vi "Periodic Tasks.vi"(8 "error in":errorcluster) -> ()   [LabVIEW 2014]
doc: "This VI runs in parallel to other tasks. It can contain as many user-defined periodic loops as you need. These can carry out PID or other sorts of timed response."
uses:
  <vilib>/Rock Robotics/WPI/Joystick/WPI_JoystickGetSetRefNum.vi
  <vilib>/Rock Robotics/WPI/RobotDrive/WPI_RobotDriveGetSetRefNum.vi
  <vilib>/Rock Robotics/Network Tables/SD Read Numeric Array.vi
  Robot Global Data.vi
  <vilib>/Rock Robotics/Network Tables/SD Write Numeric Array.vi
  <vilib>/Rock Robotics/Network Tables/SD Write Number.vi
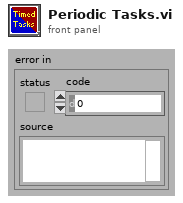
[diagram p1: front panel]
types:
  T1 = cluster{"[0]":dbl, "[1]":dbl, "[2]":dbl, "[3]":dbl, "[4]":dbl, "[5]":dbl, "[6]":dbl, "[7]":dbl, "[8]":dbl}
  T2 = typedef "WPI_JoystickDevRef.ctl" = cluster{"Device":T3}
  T3 = typedef "WPI_JoystickDeviceEnum.ctl" = enum16{"USB 0", "USB 1", "USB 2", "USB 3", "USB 4", "USB 5"}
  T4 = typedef "WPI_RobotDriveDevRef.ctl" = cluster{"DevStatus":errorcluster, "Motors[]":T5[], "Square Inputs":bool, "Max Output":dbl}
  T5 = typedef "WPI_MotorControlDeviceRef.ctl" = cluster{"DeviceStatus":errorcluster, "Type":T6, "PWM":cluster{"Controller":T7, "PWM Channel":T8, "DeadBand":T9}, "CAN":cluster{"Device Number":u8, "Control Mode":T10, "Semaphore":T11, "Max Vout":dbl, "TalonSRX Control Mode":T12}, "Invert":bool, "TransformRef":T13, "InvTransformRef":T13}
  T6 = typedef "WPI_MotorControlType.ctl" = enum16{"PWM", "CAN", "CANTalonSRX"}
  T7 = typedef "FPGA_TypedefDigitalModule.ctl" = enum16{"Controller 1"}
  T8 = typedef "FPGA_DIOPWMChannel.ctl" = enum8{"PWM 0", "PWM 1", "PWM 2", "PWM 3", "PWM 4", "PWM 5", "PWM 6", "PWM 7", "PWM 8", "PWM 9", "PWM MXP 0", "PWM MXP 1", "PWM MXP 2", "PWM MXP 3", "PWM MXP 4", "PWM MXP 5", "PWM MXP 6", "PWM MXP 7", "PWM MXP 8", "PWM MXP 9", "Invalid"}
  T9 = typedef "WPI_PWMDeadband.ctl" = cluster{"Name":string, "maxPositivePwm":i32, "minPositivePwm":i32, "centerPwm":i32, "maxNegativePwm":i32, "minNegativePwm":i32, "angularRange":u16}
  T10 = typedef "WPI_CANJaguar_ControlMode.ctl" = enum8{"Percent VBus", "Current", "Speed", "Position", "Voltage"}
  T11 = typedef "Semaphore RefNum" = refnum<k1>
  T12 = typedef "WPI_CANTalonSRX_APIControlMode.ctl" = enum8{"Percent VBus", "Speed", "Position", "Slave", "Unchanged / Invalid"}
  T13 = typedef "WPI_PWMTransform_ConPane.ctl" = refnum<vi>
  T14 = cluster{"JoystickDevRef":T2, "RobotDriveDevRef":T4}
  T15 = cluster{"X Position":dbl, "Y Position":dbl, "Angle":dbl}
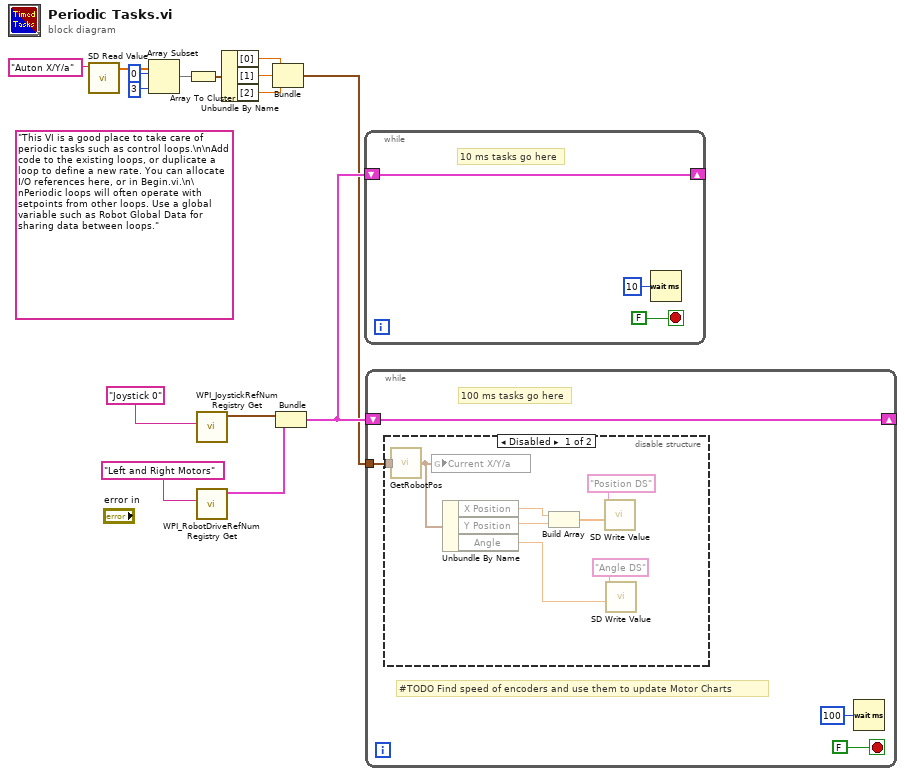
[diagram p0: block diagram]
diagram:
  (unwired) "This VI is a good place to take care of periodic tasks such as control loops.\n\nAdd code to the existing loops, or duplicate a loop to define a new rate. You can allocate I/O references here, or in Begin.vi.\n\nPeriodic loops will often operate with setpoints from other loops. Use a global variable such as Robot Global Data for sharing data between loops."
  n1 = call-poly <vilib>:"SD Read Value.vi"("Name"="Auton X/Y/a") -> ("Numeric Array"=w10:dbl[])  [unwired: 8 in, 2 out]
  n2 = Array Subset(array=w10, index=0, length=3) -> (w6:dbl[])
  n3 = Array To Cluster(array=w6) -> (cluster=w5:T1)
  n4 = call <vilib>:"WPI_JoystickRefNum Registry Get.vi"("refnum name"="Joystick 0") -> ("JoystickDevRef"=w13:T2)  [unwired: 1 in, 9 out]
  n5 = call <vilib>:"WPI_RobotDriveRefNum Registry Get.vi"("refnum name"="Left and Right Motors") -> ("RobotDriveDevRef"=w12:T4)  [unwired: 1 in, 9 out]
  n6 = Unbundle By Name(w5) -> ("[0]"=w4:dbl, "[1]"=w3:dbl, "[2]"=w2:dbl)
  n7 = Bundle("[0]"=w4, "[1]"=w3, "[2]"=w2) -> (w1:cluster{"[0]":dbl, "[1]":dbl, "[2]":dbl})  [unwired: 1 in]
  n8 = Bundle("JoystickDevRef"=w13, "RobotDriveDevRef"=w12) -> (w11:T14)  [unwired: 1 out]
  n9 = while {
    shift-right: [w16] -> _
    shift-left: w11 -> [w16]
    stop <- FALSE stop-if-true
    # "10 ms tasks go here"
    n10 = Wait (ms)(milliseconds to wait=u32 10) -> ()  [unwired: 1 out]
  }
  n11 = while {
    shift-right: [w20] -> _
    shift-left: w11 -> [w20]
    tunnel: w1 -> [w19]
    stop <- FALSE stop-if-true
    # "#TODO Find speed of encoders and use them to update Motor Charts"
    # "100 ms tasks go here"
    n12 = disable-structure shown="Disabled" {
      disable-tunnel: w19 -> [w30 _]
      frame Disabled {
        n13 = call "GetRobotPos.vi"("X/Y/a In"=w30) -> ("X/Y/a Out"=w28:T15)  [unwired: 6 in]
        n14 = global write "Robot Global Data.vi" "Current X/Y/a"(w28) -> ()
        n15 = Unbundle By Name(w28) -> ("X Position"=w27:dbl, "Y Position"=w26:dbl, "Angle"=w24:dbl)
        n16 = Build Array(w27, w26) -> (w25:dbl[])
        n17 = call-poly <vilib>:"SD Write Value.vi"("Numeric Array"=w25, "Name"="Position DS") -> ()  [unwired: 8 in, 2 out]
        n18 = call-poly <vilib>:"SD Write Value.vi"("Numeric"=w24, "Name"="Angle DS") -> ()  [unwired: 8 in, 2 out]
      }
      frame Enabled {
      }
    }
    n19 = Wait (ms)(milliseconds to wait=u32 100) -> ()  [unwired: 1 out]
  }
